vi "StringArraytoIgorWave.vi"(8 "error in (no error)":errorcluster, 10 "Wave":string[](array[string]), 11 "Name":string) -> (0 "error out":errorcluster, 3 "Igor Wave":string)   [LabVIEW 2016]
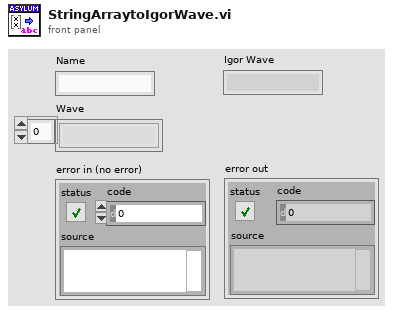
[diagram p1: front panel]
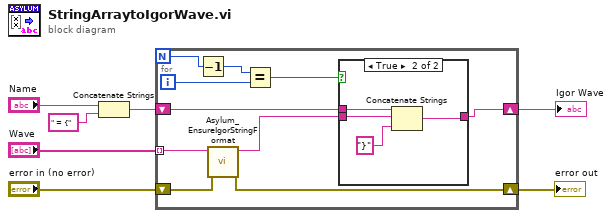
[diagram p0: block diagram]
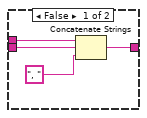
[diagram p2: hidden frame]
diagram:
  n1 = Concatenate Strings("Name", " = {" ("string")) -> (w5:string)
  n2 = for {
    N -> [w15]
    tunnel: "Wave" -> [w11] mode=indexing
    shift-right: [w16] -> w4
    shift-left: w5 -> [w17]
    shift-right: [w8] -> w2
    shift-left: "error in (no error)" -> [w9]
    i -> [w13]
    n3 = Decrement(x=w15) -> (x-1=w14:i32)
    n4 = call "Asylum_EnsureIgorStringFormat.vi"("error in (no error)"=w9, "Value"=w11) -> ("error out"=w8:errorcluster, "Value"=w10:string)  [unwired: 8 in]
    n5 = Equal?(x=w14, y=w13) -> (x = y?=w12:bool)
    n6 = case shown="True" w12 {
      tunnel: w17 -> [w21 w25]
      tunnel: w10 -> [w20 w24]
      tunnel: [w18 w22] -> w16
      frame False {
        n7 = Concatenate Strings(w21, w20, ", " ("string")) -> (w18:string)
      }
      frame True {
        n8 = Concatenate Strings(w25, w24, "}") -> (w22:string)
      }
    }
  }
  "error out" <- w2
  "Igor Wave" <- w4
